vi "SingleServiceRegistered_DiscoveryApiRoundTrip_AllNodesSucceed.vi"() -> (6 "Pass":bool, 15 "error out":errorcluster)   [LabVIEW 2020]
uses:
  Discovery_client/RPC Messages/ni_measurements_discovery_v1_RegisterServiceRequest.ctl
  Discovery_client/RPC Messages/ni_measurements_discovery_v1_ServiceDescriptor.ctl
  Discovery_client/RPC Messages/ni_measurements_discovery_v1_ServiceLocation.ctl
  Discovery_client/RPC Messages/ni_measurements_discovery_v1_EnumerateServicesRequest.ctl
  Discovery_client/RPC Messages/ni_measurements_discovery_v1_ResolveServiceRequest.ctl
  Discovery_client/Discovery_client.lvlib
panel:
  out "Register assigns registration id?":bool
  out "Unregister then enumerate lists nothing?":bool
  out "Enumerate lists service?":bool
  out "Resolve matches location?":bool
  # "Test assumes discovery service has already been started."
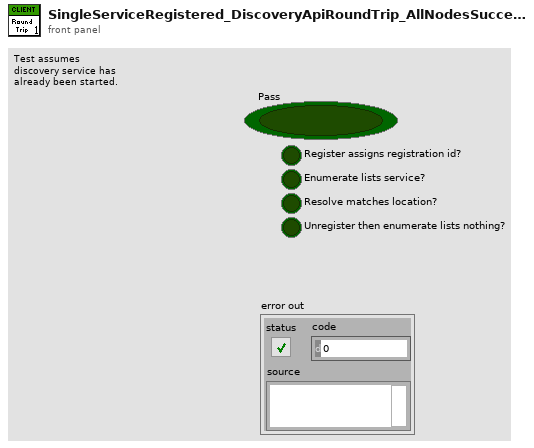
[diagram p1: front panel]
types:
  T1 = typedef "Discovery_client.lvlib/ni_measurements_discovery_v1_ResolveServiceRequest.ctl" = cluster{"provided_interface":string, "service_class":string}
  T2 = typedef "Discovery_client.lvlib/ni_measurements_discovery_v1_EnumerateServicesRequest.ctl" = cluster{"provided_interface":string}
  T3 = typedef "Discovery_client.lvlib/ni_measurements_discovery_v1_RegisterServiceRequest.ctl" = cluster{"service_description":T4, "location":T5}
  T4 = typedef "Discovery_client.lvlib/ni_measurements_discovery_v1_ServiceDescriptor.ctl" = cluster{"display_name":string, "description_url":string, "provided_interfaces":string[], "service_class":string, "attributes":string[]}
  T5 = typedef "Discovery_client.lvlib/ni_measurements_discovery_v1_ServiceLocation.ctl" = cluster{"location":string, "insecure_port":string, "ssl_authenticated_port":string}
  T6 = typedef "Discovery_client.lvlib/ni_measurements_discovery_v1_RegisterServiceResponse.ctl" = cluster{"registration_id":string}
  T7 = typedef "Discovery_client.lvlib/ni_measurements_discovery_v1_EnumerateServicesResponse.ctl" = cluster{"available_services":T4[]}
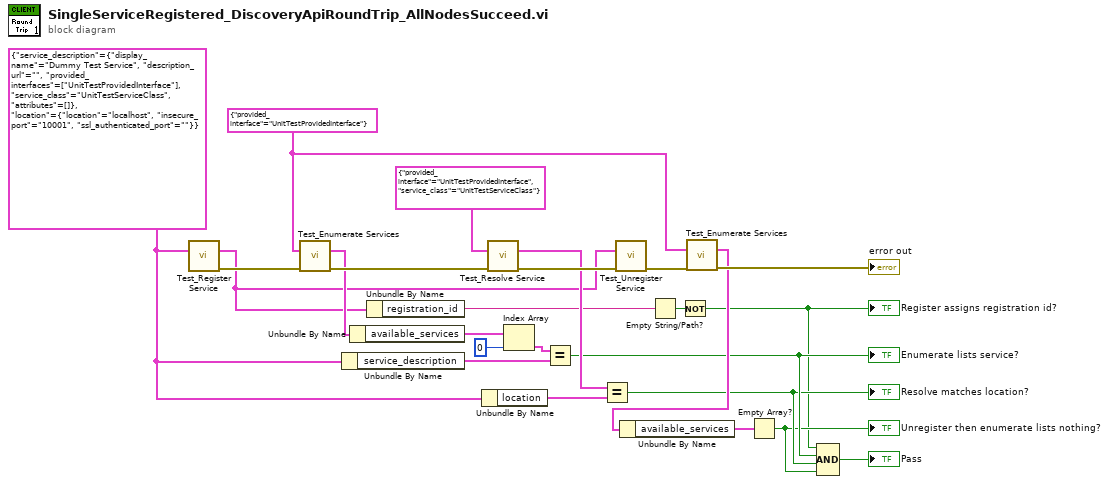
[diagram p0: block diagram]
diagram:
  w11 = T2 {"provided_interface"="UnitTestProvidedInterface"} ("Request Data")
  w17 = T3 {"service_description"={"display_name"="Dummy Test Service", "description_url"="", "provided_interfaces"=["UnitTestProvidedInterface"], "service_class"="UnitTestServiceClass", "attributes"=[]}, "location"={"location"="localhost", "insecure_port"="10001", "ssl_authenticated_port"=""}} ("Request Data")
  n1 = call "Test_Register Service.vi"("Request Data"=w17) -> ("Response Data"=w4:T6, "error out"=w25:errorcluster)  [unwired: 13 in]
  n2 = call "Test_Enumerate Services.vi"("Request Data"=w11, "error in (no error)"=w25) -> ("Response Data"=w16:T7, "error out"=w24:errorcluster)  [unwired: 12 in]
  n3 = Unbundle By Name(w17) -> ("service_description"=w15:T4)
  n4 = Unbundle By Name(w16) -> ("available_services"=w14:T4[])
  n5 = Unbundle By Name(w4) -> ("registration_id"=w3:string)
  n6 = Unbundle By Name(w17) -> ("location"=w18:T5)
  n7 = call "Test_Resolve Service.vi"("Request Data"=T1 {"provided_interface"="UnitTestProvidedInterface", "service_class"="UnitTestServiceClass"}, "error in (no error)"=w24) -> ("Response Data"=w19:T5, "error out"=w22:errorcluster)  [unwired: 12 in]
  n8 = Index Array(array=w14, index=0) -> (element=w13:T4)
  n9 = Equal?(x=w13, y=w15) -> (x = y?=w8:bool)
  "Enumerate lists service?" <- w8
  n10 = Equal?(x=w19, y=w18) -> (x = y?=w7:bool)
  "Resolve matches location?" <- w7
  n11 = call "Test_Unregister Service.vi"("Request Data"=w4, "error in (no error)"=w22) -> ("error out"=w21:errorcluster)  [unwired: 12 in, 1 out]
  n12 = Empty String/Path?(string/path=w3) -> (empty?=w2:bool)
  n13 = Not(x=w2) -> (.not. x?=w1:bool)
  "Register assigns registration id?" <- w1
  n14 = call "Test_Enumerate Services.vi"("Request Data"=w11, "error in (no error)"=w21) -> ("Response Data"=w10:T7, "error out"=→"error out":errorcluster)  [unwired: 12 in]
  n15 = Unbundle By Name(w10) -> ("available_services"=w9:T4[])
  n16 = Empty Array?(array=w9) -> (empty?=w6:bool)
  "Unregister then enumerate lists nothing?" <- w6
  n17 = Compound Arithmetic op=AND(w1, w8, w7, w6) -> (→"Pass":bool)
